vi "DevTests_Workbench.vi"() -> ()   [LabVIEW 2026]
uses:
  SDL3/Init/Init.lvlib
  SDL3/Video/Video.lvlib
  SDL3/Render/Render.lvlib
  SDL3/Pixels/PixelFormat--enum.ctl
  SDL3/Pixels/Pixels.lvlib
  SDL3/Render/TextureAccess-enum.ctl
  SDL3/Video/WindowFlags--ring.ctl
  SDL3/Init/InitFlags--ring.ctl
  SDL3/Timer/Timer.lvlib
  SDL3/Events/Events.lvlib
  SDL3/Video/WindowID--integer.ctl
  SDL3/Mouse/MouseID--integer.ctl
  SDL3/Mouse/Mouse.lvlib
  SDL3/Mouse/MouseButtonFlags--ring.ctl
  SDL3/Events/MouseMotionEventData--cluster.ctl
  SDL3/Rect/FPoint--cluster.ctl
  SDL3/Rect/Rect.lvlib
  SDL3/Video/GLAttr--enum.ctl
  SDL3/Rect/FRect--cluster.ctl
  SDL3/Blendmode/BlendMode--ring.ctl
  SDL3/Blendmode/Blendmode.lvlib
  SDL3/Keycode/Keycode--ring.ctl
  SDL3/Keycode/Keycode.lvlib
  SDL3/Video/DisplayID--integer.ctl
  SDL3/Video/DisplayMode--cluster.ctl
panel:
  out "Display Modes":T1[](array[typedef])
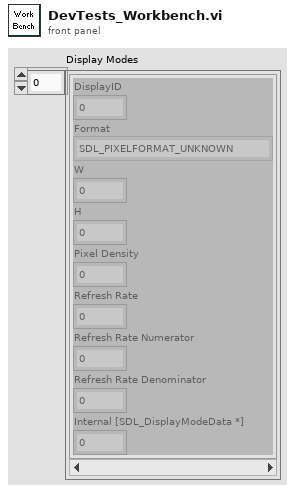
[diagram p1: front panel]
types:
  T1 = typedef "SDL3.lvlib/Video.lvlib/DisplayMode--cluster.ctl" = cluster{"DisplayID":T2, "Format":T3, "W":i32, "H":i32, "Pixel Density":sgl, "Refresh Rate":sgl, "Refresh Rate Numerator":i32, "Refresh Rate Denominator":i32, "Internal [SDL_DisplayModeData *]":i64}
  T2 = typedef "SDL3.lvlib/Video.lvlib/DisplayID--integer.ctl" = u32
  T3 = typedef "SDL3.lvlib/Pixels.lvlib/PixelFormat--enum.ctl" = enum32{"SDL_PIXELFORMAT_UNKNOWN", "SDL_PIXELFORMAT_INDEX1LSB", "SDL_PIXELFORMAT_INDEX1MSB", "SDL_PIXELFORMAT_INDEX2LSB", "SDL_PIXELFORMAT_INDEX2MSB", "SDL_PIXELFORMAT_INDEX4LSB", "SDL_PIXELFORMAT_INDEX4MSB", "SDL_PIXELFORMAT_INDEX8", "SDL_PIXELFORMAT_RGB332", "SDL_PIXELFORMAT_XRGB4444", "SDL_PIXELFORMAT_XBGR4444", "SDL_PIXELFORMAT_XRGB1555", "SDL_PIXELFORMAT_XBGR1555", "SDL_PIXELFORMAT_ARGB4444", "SDL_PIXELFORMAT_RGBA4444", "SDL_PIXELFORMAT_ABGR4444", "SDL_PIXELFORMAT_BGRA4444", "SDL_PIXELFORMAT_ARGB1555", "SDL_PIXELFORMAT_RGBA5551", "SDL_PIXELFORMAT_ABGR1555", "SDL_PIXELFORMAT_BGRA5551", "SDL_PIXELFORMAT_RGB565", "SDL_PIXELFORMAT_BGR565", "SDL_PIXELFORMAT_RGB24", "SDL_PIXELFORMAT_BGR24", "SDL_PIXELFORMAT_XRGB8888", "SDL_PIXELFORMAT_RGBX8888", "SDL_PIXELFORMAT_XBGR8888", "SDL_PIXELFORMAT_BGRX8888", "SDL_PIXELFORMAT_ARGB8888", "SDL_PIXELFORMAT_RGBA8888", "SDL_PIXELFORMAT_ABGR8888", "SDL_PIXELFORMAT_BGRA8888", "SDL_PIXELFORMAT_XRGB2101010", "SDL_PIXELFORMAT_XBGR2101010", "SDL_PIXELFORMAT_ARGB2101010", "SDL_PIXELFORMAT_ABGR2101010", "SDL_PIXELFORMAT_RGB48", "SDL_PIXELFORMAT_BGR48", "SDL_PIXELFORMAT_RGBA64", "SDL_PIXELFORMAT_ARGB64", "SDL_PIXELFORMAT_BGRA64", "SDL_PIXELFORMAT_ABGR64", "SDL_PIXELFORMAT_RGB48_FLOAT", "SDL_PIXELFORMAT_BGR48_FLOAT", "SDL_PIXELFORMAT_RGBA64_FLOAT", "SDL_PIXELFORMAT_ARGB64_FLOAT", "SDL_PIXELFORMAT_BGRA64_FLOAT", "SDL_PIXELFORMAT_ABGR64_FLOAT", "SDL_PIXELFORMAT_RGB96_FLOAT", "SDL_PIXELFORMAT_BGR96_FLOAT", "SDL_PIXELFORMAT_RGBA128_FLOAT", "SDL_PIXELFORMAT_ARGB128_FLOAT", "SDL_PIXELFORMAT_BGRA128_FLOAT", "SDL_PIXELFORMAT_ABGR128_FLOAT", "SDL_PIXELFORMAT_YV12", "SDL_PIXELFORMAT_IYUV", "SDL_PIXELFORMAT_YUY2", "SDL_PIXELFORMAT_UYVY", "SDL_PIXELFORMAT_YVYU", "SDL_PIXELFORMAT_NV12", "SDL_PIXELFORMAT_NV21", "SDL_PIXELFORMAT_P010", "SDL_PIXELFORMAT_EXTERNAL_OES"}
  T4 = typedef "SDL3.lvlib/Video.lvlib/WindowFlags--ring.ctl" = u64
  T5 = typedef "SDL3.lvlib/Blendmode.lvlib/BlendMode--ring.ctl" = u32
  T6 = typedef "SDL3.lvlib/Video.lvlib/GLAttr--enum.ctl" = enum32{"SDL_GL_RED_SIZE", "SDL_GL_GREEN_SIZE", "SDL_GL_BLUE_SIZE", "SDL_GL_ALPHA_SIZE", "SDL_GL_BUFFER_SIZE", "SDL_GL_DOUBLEBUFFER", "SDL_GL_DEPTH_SIZE", "SDL_GL_STENCIL_SIZE", "SDL_GL_ACCUM_RED_SIZE", "SDL_GL_ACCUM_GREEN_SIZE", "SDL_GL_ACCUM_BLUE_SIZE", "SDL_GL_ACCUM_ALPHA_SIZE", "SDL_GL_STEREO", "SDL_GL_MULTISAMPLEBUFFERS", "SDL_GL_MULTISAMPLESAMPLES", "SDL_GL_ACCELERATED_VISUAL", "SDL_GL_RETAINED_BACKING", "SDL_GL_CONTEXT_MAJOR_VERSION", "SDL_GL_CONTEXT_MINOR_VERSION", "SDL_GL_CONTEXT_FLAGS", "SDL_GL_CONTEXT_PROFILE_MASK", "SDL_GL_SHARE_WITH_CURRENT_CONTEXT", "SDL_GL_FRAMEBUFFER_SRGB_CAPABLE", "SDL_GL_CONTEXT_RELEASE_BEHAVIOR", "SDL_GL_CONTEXT_RESET_NOTIFICATION", "SDL_GL_CONTEXT_NO_ERROR", "SDL_GL_FLOATBUFFERS", "SDL_GL_EGL_PLATFORM"}
  T7 = enum32{"Invalid", "Standard", "Closed", "Hidden", "Minimized", "Maximized"}
  T8 = typedef "SDL3.lvlib/Events.lvlib/MouseMotionEventData--cluster.ctl" = cluster{"Timestamp":u64, "Window ID":T9, "Which":T10, "State":T11, "x":sgl, "y":sgl, "x Rel":sgl, "y Rel":sgl}
  T9 = typedef "SDL3.lvlib/Video.lvlib/WindowID--integer.ctl" = u32
  T10 = typedef "SDL3.lvlib/Mouse.lvlib/MouseID--integer.ctl" = u32
  T11 = typedef "SDL3.lvlib/Mouse.lvlib/MouseButtonFlags--ring.ctl" = u32
  T12 = typedef "SDL3.lvlib/Init.lvlib/InitFlags--ring.ctl" = u32
  T13 = typedef "SDL3.lvlib/Render.lvlib/TextureAccess-enum.ctl" = enum32{"SDL_TEXTUREACCESS_STATIC", "SDL_TEXTUREACCESS_STREAMING", "SDL_TEXTUREACCESS_TARGET"}
  T14 = typedef "SDL3.lvlib/Rect.lvlib/FPoint--cluster.ctl" = cluster{"x":sgl, "y":sgl}
  T15 = typedef "SDL3.lvlib/Rect.lvlib/FRect--cluster.ctl" = cluster{"x":sgl, "y":sgl, "w":sgl, "h":sgl}
  T16 = typedef "SDL3.lvlib/Events.lvlib/EventTypeData--enum.ctl" = enum16{"LV_NONE", "LV_UNSUPPORTED", "SDL_EVENT_QUIT", "SDL_EVENT_LOCALE_CHANGED", "SDL_EVENT_SYSTEM_THEME_CHANGED", "SDL_EVENT_DISPLAY_ORIENTATION", "SDL_EVENT_DISPLAY_ADDED", "SDL_EVENT_DISPLAY_REMOVED", "SDL_EVENT_DISPLAY_MOVED", "SDL_EVENT_DISPLAY_DESKTOP_MODE_CHANGED", "SDL_EVENT_DISPLAY_CURRENT_MODE_CHANGED", "SDL_EVENT_DISPLAY_CONTENT_SCALE_CHANGED", "SDL_EVENT_WINDOW_SHOWN", "SDL_EVENT_WINDOW_HIDDEN", "SDL_EVENT_WINDOW_EXPOSED", "SDL_EVENT_WINDOW_MOVED", "SDL_EVENT_WINDOW_RESIZED", "SDL_EVENT_WINDOW_PIXEL_SIZE_CHANGED", "SDL_EVENT_WINDOW_METAL_VIEW_RESIZED", "SDL_EVENT_WINDOW_MINIMIZED", "SDL_EVENT_WINDOW_MAXIMIZED", "SDL_EVENT_WINDOW_RESTORED", "SDL_EVENT_WINDOW_MOUSE_ENTER", "SDL_EVENT_WINDOW_MOUSE_LEAVE", "SDL_EVENT_WINDOW_FOCUS_GAINED", "SDL_EVENT_WINDOW_FOCUS_LOST", "SDL_EVENT_WINDOW_CLOSE_REQUESTED", "SDL_EVENT_WINDOW_HIT_TEST", "SDL_EVENT_WINDOW_ICCPROF_CHANGED", "SDL_EVENT_WINDOW_DISPLAY_CHANGED", "SDL_EVENT_WINDOW_DISPLAY_SCALE_CHANGED", "SDL_EVENT_WINDOW_SAFE_AREA_CHANGED", "SDL_EVENT_WINDOW_OCCLUDED", "SDL_EVENT_WINDOW_ENTER_FULLSCREEN", "SDL_EVENT_WINDOW_LEAVE_FULLSCREEN", "SDL_EVENT_WINDOW_DESTROYED", "SDL_EVENT_WINDOW_HDR_STATE_CHANGED", "SDL_EVENT_KEY_DOWN", "SDL_EVENT_KEY_UP", "SDL_EVENT_TEXT_EDITING", "SDL_EVENT_TEXT_INPUT", "SDL_EVENT_KEYMAP_CHANGED", "SDL_EVENT_KEYBOARD_ADDED", "SDL_EVENT_KEYBOARD_REMOVED", "SDL_EVENT_TEXT_EDITING_CANDIDATES", "SDL_EVENT_MOUSE_MOTION", "SDL_EVENT_MOUSE_BUTTON_DOWN", "SDL_EVENT_MOUSE_BUTTON_UP", "SDL_EVENT_MOUSE_WHEEL", "SDL_EVENT_MOUSE_ADDED", "SDL_EVENT_MOUSE_REMOVED", "SDL_EVENT_JOYSTICK_AXIS_MOTION", "SDL_EVENT_JOYSTICK_BALL_MOTION", "SDL_EVENT_JOYSTICK_HAT_MOTION", "SDL_EVENT_JOYSTICK_BUTTON_DOWN", "SDL_EVENT_JOYSTICK_BUTTON_UP", "SDL_EVENT_JOYSTICK_ADDED", "SDL_EVENT_JOYSTICK_REMOVED", "SDL_EVENT_JOYSTICK_BATTERY_UPDATED", "SDL_EVENT_JOYSTICK_UPDATE_COMPLETE", "SDL_EVENT_GAMEPAD_AXIS_MOTION", "SDL_EVENT_GAMEPAD_BUTTON_DOWN", "SDL_EVENT_GAMEPAD_BUTTON_UP", "SDL_EVENT_GAMEPAD_ADDED", "SDL_EVENT_GAMEPAD_REMOVED", "SDL_EVENT_GAMEPAD_REMAPPED", "SDL_EVENT_GAMEPAD_TOUCHPAD_DOWN", "SDL_EVENT_GAMEPAD_TOUCHPAD_MOTION", "SDL_EVENT_GAMEPAD_TOUCHPAD_UP", "SDL_EVENT_GAMEPAD_SENSOR_UPDATE", "SDL_EVENT_GAMEPAD_UPDATE_COMPLETE", "SDL_EVENT_GAMEPAD_STEAM_HANDLE_UPDATED", "SDL_EVENT_FINGER_DOWN", "SDL_EVENT_FINGER_UP", "SDL_EVENT_FINGER_MOTION", "SDL_EVENT_CLIPBOARD_UPDATE", "SDL_EVENT_DROP_FILE", "SDL_EVENT_DROP_TEXT", "SDL_EVENT_DROP_BEGIN", "SDL_EVENT_DROP_COMPLETE", "SDL_EVENT_DROP_POSITION", "SDL_EVENT_AUDIO_DEVICE_ADDED", "SDL_EVENT_AUDIO_DEVICE_REMOVED", "SDL_EVENT_AUDIO_DEVICE_FORMAT_CHANGED", "SDL_EVENT_SENSOR_UPDATE", "SDL_EVENT_PEN_PROXIMITY_IN", "SDL_EVENT_PEN_PROXIMITY_OUT", "SDL_EVENT_PEN_DOWN", "SDL_EVENT_PEN_UP", "SDL_EVENT_PEN_BUTTON_DOWN", "SDL_EVENT_PEN_BUTTON_UP", "SDL_EVENT_PEN_MOTION", "SDL_EVENT_PEN_AXIS", "SDL_EVENT_CAMERA_DEVICE_ADDED", "SDL_EVENT_CAMERA_DEVICE_REMOVED", "SDL_EVENT_CAMERA_DEVICE_APPROVED", "SDL_EVENT_CAMERA_DEVICE_DENIED", "SDL_EVENT_RENDER_TARGETS_RESET", "SDL_EVENT_RENDER_DEVICE_RESET", "SDL_EVENT_POLL_SENTINEL", "SDL_EVENT_USER"}
  T17 = typedef "SDL3.lvlib/Events.lvlib/MouseMotionEvent--cluster.ctl" = cluster{"Timestamp":u64, "Window ID":T9, "Which":T10, "State":T11, "x":sgl, "y":sgl, "x Rel":sgl, "y Rel":sgl}
  T18 = typedef "SDL3.lvlib/Keycode.lvlib/Keycode--ring.ctl" = u32
  T19 = typedef "SDL3.lvlib/Events.lvlib/KeyboardEventData--cluster.ctl" = cluster{"Timestamp":u64, "Window ID":T9, "Which":T20, "Scancode":T21, "Key":T18, "Mod":T22, "Raw":u16, "Down":bool, "Repeat":bool}
  T20 = typedef "SDL3.lvlib/Keyboard.lvlib/KeyboardID--integer.ctl" = u32
  T21 = typedef "SDL3.lvlib/Events.lvlib/Scancode--integer.ctl" = u32
  T22 = typedef "SDL3.lvlib/Keycode.lvlib/Keymod--ring.ctl" = u16
  T23 = typedef "SDL3.lvlib/Render.lvlib/Vertex--cluster.ctl" = cluster{"Position":T14, "Color":T24, "TexCoord":T14}
  T24 = typedef "SDL3.lvlib/Pixels.lvlib/FColor--cluster.ctl" = cluster{"r":sgl, "g":sgl, "b":sgl, "a":sgl}
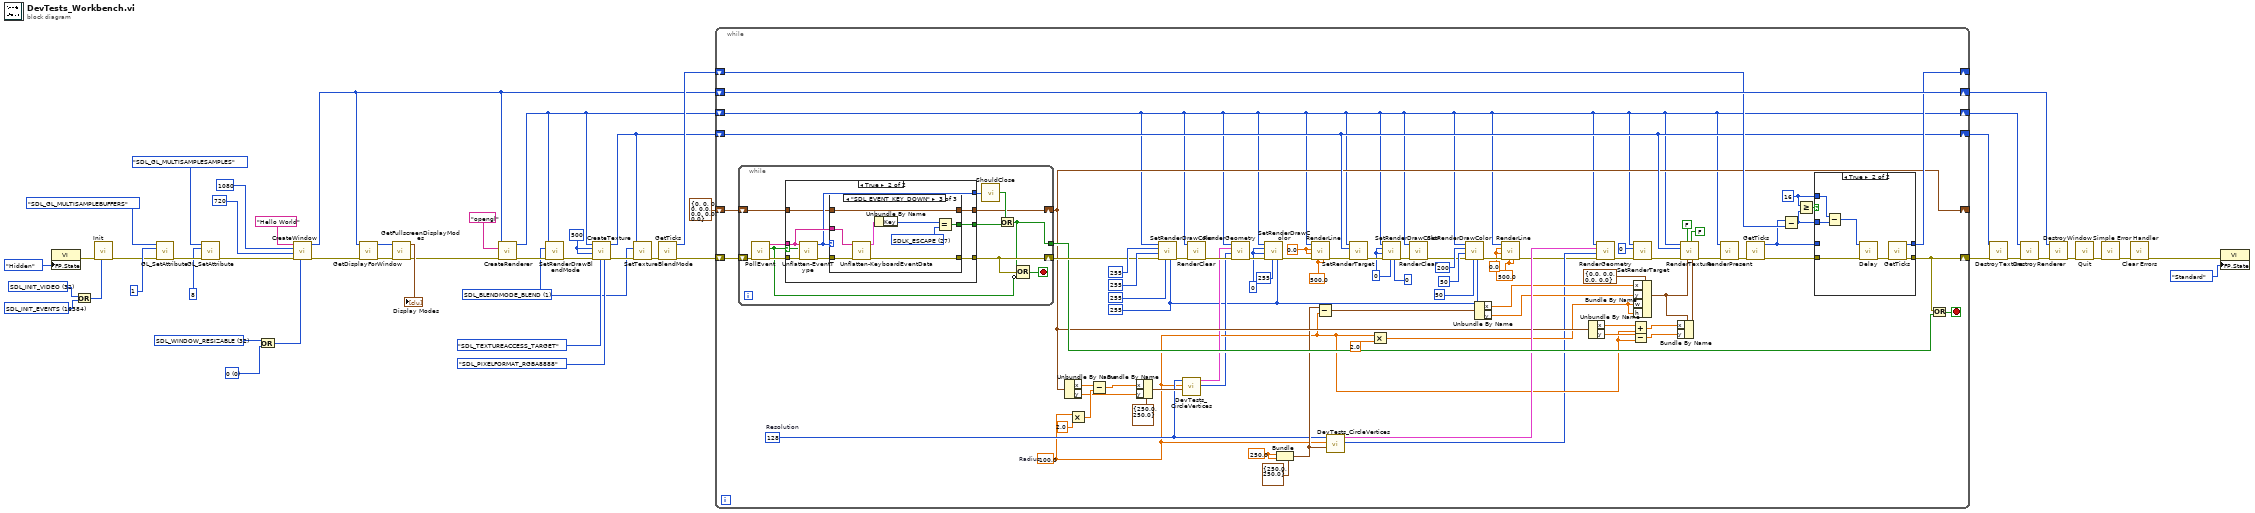
[diagram p0: block diagram]
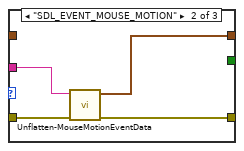
[diagram p4: hidden frame]
diagram:
  w10 = T4 0 items=["0"=0, "SDL_WINDOW_FULLSCREEN"=1, "SDL_WINDOW_OPENGL"=2, "SDL_WINDOW_OCCLUDED"=4, "SDL_WINDOW_HIDDEN"=8, "SDL_WINDOW_BORDERLESS"=16, "SDL_WINDOW_RESIZABLE"=32, "SDL_WINDOW_MINIMIZED"=64, "SDL_WINDOW_MAXIMIZED"=128, "SDL_WINDOW_MOUSE_GRABBED"=256, "SDL_WINDOW_INPUT_FOCUS"=512, "SDL_WINDOW_MOUSE_FOCUS"=1024, "SDL_WINDOW_EXTERNAL"=2048, "SDL_WINDOW_MODAL"=4096, "SDL_WINDOW_HIGH_PIXEL_DENSITY"=8192, "SDL_WINDOW_MOUSE_CAPTURE"=16384, "SDL_WINDOW_MOUSE_RELATIVE_MODE"=32768, "SDL_WINDOW_ALWAYS_ON_TOP"=65536, "SDL_WINDOW_UTILITY"=131072, "SDL_WINDOW_TOOLTIP"=262144, "SDL_WINDOW_POPUP_MENU"=524288, "SDL_WINDOW_KEYBOARD_GRABBED"=1048576, "SDL_WINDOW_VULKAN"=268435456, "SDL_WINDOW_METAL"=536870912, "SDL_WINDOW_TRANSPARENT"=1073741824, "SDL_WINDOW_NOT_FOCUSABLE"=2147483648] ("y")
  w7 = T5 1 items=["SDL_BLENDMODE_NONE"=0, "SDL_BLENDMODE_BLEND"=1, "SDL_BLENDMODE_BLEND_PREMULTIPLIED"=16, "SDL_BLENDMODE_ADD"=2, "SDL_BLENDMODE_ADD_PREMULTIPLIED"=32, "SDL_BLENDMODE_MOD"=4, "SDL_BLENDMODE_MUL"=8, "SDL_BLENDMODE_INVALID"=2147483647] ("Blend Mode")
  w25 = T12 16384 items=["NONE"=0, "SDL_INIT_AUDIO"=16, "SDL_INIT_VIDEO"=32, "SDL_INIT_JOYSTICK"=512, "SDL_INIT_HAPTIC"=4096, "SDL_INIT_GAMEPAD"=8192, "SDL_INIT_EVENTS"=16384, "SDL_INIT_SENSOR"=32768, "SDL_INIT_CAMER"=65536] ("y")
  w29 = T12 32 items=["NONE"=0, "SDL_INIT_AUDIO"=16, "SDL_INIT_VIDEO"=32, "SDL_INIT_JOYSTICK"=512, "SDL_INIT_HAPTIC"=4096, "SDL_INIT_GAMEPAD"=8192, "SDL_INIT_EVENTS"=16384, "SDL_INIT_SENSOR"=32768, "SDL_INIT_CAMER"=65536] ("InitFlags")
  w43 = 500 ("w")
  w47 = T4 32 items=["0"=0, "SDL_WINDOW_FULLSCREEN"=1, "SDL_WINDOW_OPENGL"=2, "SDL_WINDOW_OCCLUDED"=4, "SDL_WINDOW_HIDDEN"=8, "SDL_WINDOW_BORDERLESS"=16, "SDL_WINDOW_RESIZABLE"=32, "SDL_WINDOW_MINIMIZED"=64, "SDL_WINDOW_MAXIMIZED"=128, "SDL_WINDOW_MOUSE_GRABBED"=256, "SDL_WINDOW_INPUT_FOCUS"=512, "SDL_WINDOW_MOUSE_FOCUS"=1024, "SDL_WINDOW_EXTERNAL"=2048, "SDL_WINDOW_MODAL"=4096, "SDL_WINDOW_HIGH_PIXEL_DENSITY"=8192, "SDL_WINDOW_MOUSE_CAPTURE"=16384, "SDL_WINDOW_MOUSE_RELATIVE_MODE"=32768, "SDL_WINDOW_ALWAYS_ON_TOP"=65536, "SDL_WINDOW_UTILITY"=131072, "SDL_WINDOW_TOOLTIP"=262144, "SDL_WINDOW_POPUP_MENU"=524288, "SDL_WINDOW_KEYBOARD_GRABBED"=1048576, "SDL_WINDOW_VULKAN"=268435456, "SDL_WINDOW_METAL"=536870912, "SDL_WINDOW_TRANSPARENT"=1073741824, "SDL_WINDOW_NOT_FOCUSABLE"=2147483648] ("flags (0)")
  n1 = property class="VI"("FP.State"=T7."Hidden" ("Front Panel Window:State")) -> (error out=w34:errorcluster)  [unwired: 2 in, 1 out]
  n2 = Or(x=w29, y=w25) -> (x .or. y?=w26:T12)
  n3 = call "Init.vi"("InitFlags"=w26, "No Error"=w34) -> ("error out"=w13:errorcluster)  [unwired: 9 in]
  n4 = call "GL_SetAttribute.vi"("No Error"=w13, "Value"=1, "GL Attribute"=GLAttr--enum."SDL_GL_MULTISAMPLEBUFFERS") -> ("Error Out"=w21:errorcluster)  [unwired: 8 in]
  n5 = call "GL_SetAttribute.vi"("No Error"=w21, "Value"=8, "GL Attribute"=GLAttr--enum."SDL_GL_MULTISAMPLESAMPLES") -> ("Error Out"=w22:errorcluster)  [unwired: 8 in]
  n6 = Compound Arithmetic op=OR(w47, w10) -> (w11:T4)
  n7 = call "CreateWindow.vi"("Flags (0)"=w11, "No Error"=w22, "h"=720, "w"=1080, "Title"="Hello World" ("title")) -> ("Error Out"=w6:errorcluster, "Window [SDL_Window *]"=w5:i64)  [unwired: 5 in]
  n8 = call "GetDisplayForWindow.vi"("No Error"=w6, "Window [SDL_Window *]"=w5) -> ("Error Out"=w4:errorcluster, "DisplayID"=w3:T2)  [unwired: 8 in]
  n9 = call "GetFullscreenDisplayModes.vi"("No Error"=w4, "DisplayID"=w3) -> ("Error Out"=w1:errorcluster, "Display Modes"=→"Display Modes":T1[])  [unwired: 8 in]
  n10 = call "CreateRenderer.vi"("No Error"=w1, "Name (\"\": NULL)"="opengl" ("Name (\"\": NULL)"), "Window [SDL_Window *]"=w5) -> ("Error Out"=w44:errorcluster, "Renderer [SDL_Renderer *]"=w8:i64)  [unwired: 7 in]
  n11 = call "SetRenderDrawBlendMode.vi"("No Error"=w44, "Blend Mode"=w7, "Renderer [SDL_Renderer *]"=w8) -> ("error out"=w9:errorcluster)  [unwired: 8 in]
  n12 = call "CreateTexture.vi"("Pixel Format"=PixelFormat--enum."SDL_PIXELFORMAT_RGBA8888" ("pixel_format"), "Texture Access"=TextureAccess-enum."SDL_TEXTUREACCESS_TARGET" ("texture_access"), "No Error"=w9, "h"=w43, "w"=w43, "Renderer [SDL_Renderer *]"=w8) -> ("error out"=w16:errorcluster, "Texture [SDL_Texture *]"=w14:i64)  [unwired: 4 in]
  n13 = call "SetTextureBlendMode.vi"("No Error"=w16, "Blend Mode"=w7, "Texture [SDL_Texture *]"=w14) -> ("error out"=w15:errorcluster)  [unwired: 8 in]
  n14 = call "GetTicks.vi"("No Error"=w15) -> ("error out"=w28:errorcluster, "Ticks [ms]"=w27:u64)  [unwired: 9 in]
  n15 = while {
    shift-right: [w98] -> w37
    shift-left: w14 -> [w98]
    shift-right: [w53] -> w38
    shift-left: w8 -> [w53]
    shift-right: [w126] -> w39
    shift-left: w5 -> [w126]
    shift-right: [w100] -> w46
    shift-left: w28 -> [w106]
    shift-right: [w114] -> _
    shift-left: w27 -> [w111]
    shift-right: [w97] -> _
    shift-left: T8 {"Timestamp"=0, "Window ID"=0, "Which"=0, "State"=0, "x"=0.0, "y"=0.0, "x Rel"=0.0, "y Rel"=0.0} ("MouseMotionEvent") -> [w105]
    stop <- w101 stop-if-true
    w51 = sgl 500.0 ("X2")
    w52 = sgl 0.0 ("X1")
    w57 = u8 0 ("R")
    w61 = sgl 0.0 ("X1")
    w62 = sgl 500.0 ("X2")
    w66 = u8 0 ("r")
    w84 = sgl 250.0 ("x")
    w71 = sgl 100.0  # Radius
    w77 = 128  # Resolution
    w110 = u64 16
    w58 = u8 255 ("a")
    n16 = while {
      shift-right: [w129] -> w104
      shift-left: w106 -> [w138]
      tunnel: [w128] -> w102
      shift-right: [w131] -> w97
      shift-left: w105 -> [w130]
      stop <- w137 stop-if-true
      n17 = call "PollEvent.vi"("No Error"=w138) -> ("error out"=w136:errorcluster, "Event Occured?"=w134:bool, "Event Binary Data"=w135:string)  [unwired: 8 in]
      n18 = case shown="True" w134 {
        tunnel: w136 -> [w140 w148]
        tunnel: w135 -> [_ w147]
        tunnel: [w140 w144] -> w129
        tunnel: [_ w146] -> w133
        tunnel: [w139 w143] -> w131
        tunnel: w130 -> [w139 w142]
        tunnel: [_ w141] -> w127
        frame False {
        }
        frame True {
          n19 = call "Unflatten-EventType.vi"("error in (no error)"=w148, "Event Binary Data In"=w147) -> ("error out"=w145:errorcluster, "EventType"=w146:T16)  [unwired: 8 in]
          n20 = case shown="\"SDL_EVENT_KEY_DOWN\"" w146 {
            tunnel: w147 -> [_ w153 w160]
            tunnel: w145 -> [w150 w154 w161]
            tunnel: [w150 w152 w159] -> w144
            tunnel: [w149 w151 w162] -> w143
            tunnel: w142 -> [w149 _ w162]
            tunnel: [_ _ w155] -> w141
            frame Default {
            }
            frame "SDL_EVENT_MOUSE_MOTION" {
              n21 = call "Unflatten-MouseMotionEventData.vi"("error in (no error)"=w154, "Event Binary Data"=w153) -> ("error out"=w152:errorcluster, "Event Data"=w151:T17)  [unwired: 8 in]
            }
            frame "SDL_EVENT_KEY_DOWN" {
              w156 = T18 27 items=["SDLK_SCANCODE_MASK"=1073741824, "SDLK_UNKNOWN"=0, "SDLK_RETURN"=13, "SDLK_ESCAPE"=27, "SDLK_BACKSPACE"=8, "SDLK_TAB"=9, "SDLK_SPACE"=32, "SDLK_EXCLAIM"=33, "SDLK_DBLAPOSTROPHE"=34, "SDLK_HASH"=35, "SDLK_DOLLAR"=36, "SDLK_PERCENT"=37, "SDLK_AMPERSAND"=38, "SDLK_APOSTROPHE"=39, "SDLK_LEFTPAREN"=40, "SDLK_RIGHTPAREN"=41, "SDLK_ASTERISK"=42, "SDLK_PLUS"=43, "SDLK_COMMA"=44, "SDLK_MINUS"=45, "SDLK_PERIOD"=46, "SDLK_SLASH"=47, "SDLK_0"=48, "SDLK_1"=49, "SDLK_2"=50, "SDLK_3"=51, "SDLK_4"=52, "SDLK_5"=53, "SDLK_6"=54, "SDLK_7"=55, "SDLK_8"=56, "SDLK_9"=57, "SDLK_COLON"=58, "SDLK_SEMICOLON"=59, "SDLK_LESS"=60, "SDLK_EQUALS"=61, "SDLK_GREATER"=62, "SDLK_QUESTION"=63, "SDLK_AT"=64, "SDLK_LEFTBRACKET"=91, "SDLK_BACKSLASH"=92, "SDLK_RIGHTBRACKET"=93, "SDLK_CARET"=94, "SDLK_UNDERSCORE"=95, "SDLK_GRAVE"=96, "SDLK_A"=97, "SDLK_B"=98, "SDLK_C"=99, "SDLK_D"=100, "SDLK_E"=101, "SDLK_F"=102, "SDLK_G"=103, "SDLK_H"=104, "SDLK_I"=105, "SDLK_J"=106, "SDLK_K"=107, "SDLK_L"=108, "SDLK_M"=109, "SDLK_N"=110, "SDLK_O"=111, "SDLK_P"=112, "SDLK_Q"=113, "SDLK_R"=114, "SDLK_S"=115, "SDLK_T"=116, "SDLK_U"=117, "SDLK_V"=118, "SDLK_W"=119, "SDLK_X"=120, "SDLK_Y"=121, "SDLK_Z"=122, "SDLK_LEFTBRACE"=123, "SDLK_PIPE"=124, "SDLK_RIGHTBRACE"=125, "SDLK_TILDE"=126, "SDLK_DELETE"=127, "SDLK_PLUSMINUS"=177, "SDLK_CAPSLOCK"=1073741881, "SDLK_F1"=1073741882, "SDLK_F2"=1073741883, "SDLK_F3"=1073741884, "SDLK_F4"=1073741885, "SDLK_F5"=1073741886, "SDLK_F6"=1073741887, "SDLK_F7"=1073741888, "SDLK_F8"=1073741889, "SDLK_F9"=1073741890, "SDLK_F10"=1073741891, "SDLK_F11"=1073741892, "SDLK_F12"=1073741893, "SDLK_PRINTSCREEN"=1073741894, "SDLK_SCROLLLOCK"=1073741895, "SDLK_PAUSE"=1073741896, "SDLK_INSERT"=1073741897, "SDLK_HOME"=1073741898, "SDLK_PAGEUP"=1073741899, "SDLK_END"=1073741901, "SDLK_PAGEDOWN"=1073741902, "SDLK_RIGHT"=1073741903, "SDLK_LEFT"=1073741904, "SDLK_DOWN"=1073741905, "SDLK_UP"=1073741906, "SDLK_NUMLOCKCLEAR"=1073741907, "SDLK_KP_DIVIDE"=1073741908, "SDLK_KP_MULTIPLY"=1073741909, "SDLK_KP_MINUS"=1073741910, "SDLK_KP_PLUS"=1073741911, "SDLK_KP_ENTER"=1073741912, "SDLK_KP_1"=1073741913, "SDLK_KP_2"=1073741914, "SDLK_KP_3"=1073741915, "SDLK_KP_4"=1073741916, "SDLK_KP_5"=1073741917, "SDLK_KP_6"=1073741918, "SDLK_KP_7"=1073741919, "SDLK_KP_8"=1073741920, "SDLK_KP_9"=1073741921, "SDLK_KP_0"=1073741922, "SDLK_KP_PERIOD"=1073741923, "SDLK_APPLICATION"=1073741925, "SDLK_POWER"=1073741926, "SDLK_KP_EQUALS"=1073741927, "SDLK_F13"=1073741928, "SDLK_F14"=1073741929, "SDLK_F15"=1073741930, "SDLK_F16"=1073741931, "SDLK_F17"=1073741932, "SDLK_F18"=1073741933, "SDLK_F19"=1073741934, "SDLK_F20"=1073741935, "SDLK_F21"=1073741936, "SDLK_F22"=1073741937, "SDLK_F23"=1073741938, "SDLK_F24"=1073741939, "SDLK_EXECUTE"=1073741940, "SDLK_HELP"=1073741941, "SDLK_MENU"=1073741942, "SDLK_SELECT"=1073741943, "SDLK_STOP"=1073741944, "SDLK_AGAIN"=1073741945, "SDLK_UNDO"=1073741946, "SDLK_CUT"=1073741947, "SDLK_COPY"=1073741948, "SDLK_PASTE"=1073741949, "SDLK_FIND"=1073741950, "SDLK_MUTE"=1073741951, "SDLK_VOLUMEUP"=1073741952, "SDLK_VOLUMEDOWN"=1073741953, "SDLK_KP_COMMA"=1073741957, "SDLK_KP_EQUALSAS400"=1073741958, "SDLK_ALTERASE"=1073741977, "SDLK_SYSREQ"=1073741978, "SDLK_CANCEL"=1073741979, "SDLK_CLEAR"=1073741980, "SDLK_PRIOR"=1073741981, "SDLK_RETURN2"=1073741982, "SDLK_SEPARATOR"=1073741983, "SDLK_OUT"=1073741984, "SDLK_OPER"=1073741985, "SDLK_CLEARAGAIN"=1073741986, "SDLK_CRSEL"=1073741987, "SDLK_EXSEL"=1073741988, "SDLK_KP_00"=1073742000, "SDLK_KP_000"=1073742001, "SDLK_THOUSANDSSEPARATOR"=1073742002, "SDLK_DECIMALSEPARATOR"=1073742003, "SDLK_CURRENCYUNIT"=1073742004, "SDLK_CURRENCYSUBUNIT"=1073742005, "SDLK_KP_LEFTPAREN"=1073742006, "SDLK_KP_RIGHTPAREN"=1073742007, "SDLK_KP_LEFTBRACE"=1073742008, "SDLK_KP_RIGHTBRACE"=1073742009, "SDLK_KP_TAB"=1073742010, "SDLK_KP_BACKSPACE"=1073742011, "SDLK_KP_A"=1073742012, "SDLK_KP_B"=1073742013, "SDLK_KP_C"=1073742014, "SDLK_KP_D"=1073742015, "SDLK_KP_E"=1073742016, "SDLK_KP_F"=1073742017, "SDLK_KP_XOR"=1073742018, "SDLK_KP_POWER"=1073742019, "SDLK_KP_PERCENT"=1073742020, "SDLK_KP_LESS"=1073742021, "SDLK_KP_GREATER"=1073742022, "SDLK_KP_AMPERSAND"=1073742023, "SDLK_KP_DBLAMPERSAND"=1073742024, "SDLK_KP_VERTICALBAR"=1073742025, "SDLK_KP_DBLVERTICALBAR"=1073742026, "SDLK_KP_COLON"=1073742027, "SDLK_KP_HASH"=1073742028, "SDLK_KP_SPACE"=1073742029, "SDLK_KP_AT"=1073742030, "SDLK_KP_EXCLAM"=1073742031, "SDLK_KP_MEMSTORE"=1073742032, "SDLK_KP_MEMRECALL"=1073742033, "SDLK_KP_MEMCLEAR"=1073742034, "SDLK_KP_MEMADD"=1073742035, "SDLK_KP_MEMSUBTRACT"=1073742036, "SDLK_KP_MEMMULTIPLY"=1073742037, "SDLK_KP_MEMDIVIDE"=1073742038, "SDLK_KP_PLUSMINUS"=1073742039, "SDLK_KP_CLEAR"=1073742040, "SDLK_KP_CLEARENTRY"=1073742041, "SDLK_KP_BINARY"=1073742042, "SDLK_KP_OCTAL"=1073742043, "SDLK_KP_DECIMAL"=1073742044, "SDLK_KP_HEXADECIMAL"=1073742045, "SDLK_LCTRL"=1073742048, "SDLK_LSHIFT"=1073742049, "SDLK_LALT"=1073742050, "SDLK_LGUI"=1073742051, "SDLK_RCTRL"=1073742052, "SDLK_RSHIFT"=1073742053, "SDLK_RALT"=1073742054, "SDLK_RGUI"=1073742055, "SDLK_MODE"=1073742081, "SDLK_SLEEP"=1073742082, "SDLK_WAKE"=1073742083, "SDLK_CHANNEL_INCREMENT"=1073742084, "SDLK_CHANNEL_DECREMENT"=1073742085, "SDLK_MEDIA_PLAY"=1073742086, "SDLK_MEDIA_PAUSE"=1073742087, "SDLK_MEDIA_RECORD"=1073742088, "SDLK_MEDIA_FAST_FORWARD"=1073742089, "SDLK_MEDIA_REWIND"=1073742090, "SDLK_MEDIA_NEXT_TRACK"=1073742091, "SDLK_MEDIA_PREVIOUS_TRACK"=1073742092, "SDLK_MEDIA_STOP"=1073742093, "SDLK_MEDIA_EJECT"=1073742094, "SDLK_MEDIA_PLAY_PAUSE"=1073742095, "SDLK_MEDIA_SELECT"=1073742096, "SDLK_AC_NEW"=1073742097, "SDLK_AC_OPEN"=1073742098, "SDLK_AC_CLOSE"=1073742099, "SDLK_AC_EXIT"=1073742100, "SDLK_AC_SAVE"=1073742101, "SDLK_AC_PRINT"=1073742102, "SDLK_AC_PROPERTIES"=1073742103, "SDLK_AC_SEARCH"=1073742104, "SDLK_AC_HOME"=1073742105, "SDLK_AC_BACK"=1073742106, "SDLK_AC_FORWARD"=1073742107, "SDLK_AC_STOP"=1073742108, "SDLK_AC_REFRESH"=1073742109, "SDLK_AC_BOOKMARKS"=1073742110, "SDLK_SOFTLEFT"=1073742111, "SDLK_SOFTRIGHT"=1073742112, "SDLK_CALL"=1073742113, "SDLK_ENDCALL"=1073742114] ("y")
              n22 = call "Unflatten-KeyboardEventData.vi"("error in (no error)"=w161, "Event Binary Data"=w160) -> ("error out"=w159:errorcluster, "Event Data"=w158:T19)  [unwired: 8 in]
              n23 = Unbundle By Name(w158) -> ("Key"=w157:T18)
              n24 = Equal?(x=w157, y=w156) -> (x = y?=w155:bool)
            }
          }
        }
      }
      n25 = call "ShouldClose.vi"("EventType"=w133) -> ("Close?"=w132:bool)
      n26 = Or(x=w132, y=w127) -> (x .or. y?=w128:bool)
      n27 = Compound Arithmetic op=OR(w128, w129, invert w134) -> (w137:bool)
    }
    n28 = Unbundle By Name(w97) -> ("x"=w79:sgl, "y"=w72:sgl)
    n29 = Multiply(x=w71, y=sgl 2.0) -> (x*y=w74:sgl)
    n30 = Subtract(x=w79, y=w74) -> (x-y=w75:sgl)
    n31 = Bundle By Name(cluster=T14 {"x"=250.0, "y"=250.0} ("Center"), "x"=w75, "y"=w72) -> (w78:T14)
    n32 = call "SetRenderDrawColor.vi"("a"=w58, "b"=u8 255, "No Error"=w104, "g"=u8 255, "r"=u8 255, "Renderer [SDL_Renderer *]"=w53) -> ("error out"=w123:errorcluster)  [unwired: 5 in]
    n33 = call "DevTests_CircleVertices.vi"("Center"=w78, "Radius"=w71, "Quality"=w77) -> ("Draw Order"=w70:i32[], "Vertices"=w76:T23[])  [unwired: 7 in]
    n34 = call "RenderClear.vi"("No Error"=w123, "Renderer [SDL_Renderer *]"=w53) -> ("error out"=w81:errorcluster)  [unwired: 9 in]
    n35 = call "RenderGeometry.vi"("No Error"=w81, "Indices (Empty)"=w70, "Vertices"=w76, "Renderer [SDL_Renderer *]"=w53) -> ("error out"=w59:errorcluster)  [unwired: 7 in]
    n36 = call "SetRenderDrawColor.vi"("a"=w58, "b"=u8 255 ("B"), "No Error"=w59, "g"=w57, "r"=w57, "Renderer [SDL_Renderer *]"=w53) -> ("error out"=w55:errorcluster)  [unwired: 5 in]
    n37 = Bundle(cluster=T14 {"x"=250.0, "y"=250.0} ("Center"), "x"=w84, "y"=w84) -> (w83:T14)
    n38 = call "RenderLine.vi"("y2"=w62, "x2"=w62, "No Error"=w55, "y1"=w61, "x1"=w61, "Renderer [SDL_Renderer *]"=w53) -> ("error out"=w60:errorcluster)  [unwired: 5 in]
    n39 = Subtract(x=w83, y=w71) -> (x-y=w90:T14)
    n40 = call "DevTests_CircleVertices.vi"("Center"=w83, "Radius"=w71, "Quality"=w77) -> ("Draw Order"=w69:i32[], "Vertices"=w99:T23[])  [unwired: 7 in]
    n41 = call "SetRenderTarget.vi"("No Error"=w60, "Texture [SDL_Texture *]"=w98, "Renderer [SDL_Renderer *]"=w53) -> ("error out"=w68:errorcluster)  [unwired: 8 in]
    n42 = Multiply(x=w71, y=sgl 2.0) -> (x*y=w85:sgl)
    n43 = call "SetRenderDrawColor.vi"("a"=u8 0 ("A"), "b"=w66, "No Error"=w68, "g"=w66, "r"=w66, "Renderer [SDL_Renderer *]"=w53) -> ("error out"=w67:errorcluster)  [unwired: 5 in]
    n44 = call "RenderClear.vi"("No Error"=w67, "Renderer [SDL_Renderer *]"=w53) -> ("error out"=w103:errorcluster)  [unwired: 9 in]
    n45 = call "SetRenderDrawColor.vi"("a"=w58, "b"=u8 50, "No Error"=w103, "g"=u8 50, "r"=u8 200, "Renderer [SDL_Renderer *]"=w53) -> ("error out"=w54:errorcluster)  [unwired: 5 in]
    n46 = Unbundle By Name(w90) -> ("x"=w89:sgl, "y"=w88:sgl)
    n47 = call "RenderLine.vi"("y2"=w51, "x2"=w51, "No Error"=w54, "y1"=w52, "x1"=w52, "Renderer [SDL_Renderer *]"=w53) -> ("error out"=w50:errorcluster)  [unwired: 5 in]
    n48 = Unbundle By Name(w97) -> ("x"=w95:sgl, "y"=w94:sgl)
    n49 = call "RenderGeometry.vi"("No Error"=w50, "Indices (Empty)"=w69, "Vertices"=w99, "Renderer [SDL_Renderer *]"=w53) -> ("error out"=w115:errorcluster)  [unwired: 7 in]
    n50 = Add(x=w95, y=w71) -> (x+y=w93:sgl)
    n51 = Subtract(x=w94, y=w71) -> (x-y=w92:sgl)
    n52 = Bundle By Name(cluster=T15 {"x"=0.0, "y"=0.0, "w"=0.0, "h"=0.0} ("Srcrect"), "x"=w89, "y"=w88, "w"=w85, "h"=w85) -> (w87:T15)
    n53 = call "SetRenderTarget.vi"("No Error"=w115, "Texture [SDL_Texture *]"=i64 0 ("texture [SDL_Texture *]"), "Renderer [SDL_Renderer *]"=w53) -> ("error out"=w124:errorcluster)  [unwired: 8 in]
    n54 = Bundle By Name(cluster=w87, "x"=w93, "y"=w92) -> (w96:T15)
    n55 = call "RenderTexture.vi"("Dstrect"=w96, "Entire Rendering Target (F)"=FALSE, "Srcrect"=w87, "Entire Texture (F)"=FALSE, "No Error"=w124, "Texture [SDL_Texture *]"=w98, "Renderer [SDL_Renderer *]"=w53) -> ("error out"=w125:errorcluster)  [unwired: 4 in]
    n56 = call "RenderPresent.vi"("No Error"=w125, "Renderer [SDL_Renderer *]"=w53) -> ("error out"=w113:errorcluster)  [unwired: 9 in]
    n57 = call "GetTicks.vi"("No Error"=w113) -> ("error out"=w112:errorcluster, "Ticks [ms]"=w107:u64)  [unwired: 9 in]
    n58 = Subtract(x=w107, y=w111) -> (x-y=w109:u64)
    n59 = Greater Or Equal?(x=w110, y=w109) -> (x >= y?=w108:bool)
    n60 = case shown="True" w108 {
      tunnel: [w163 w171] -> w100
      tunnel: [w164 w170] -> w114
      tunnel: w112 -> [w163 w169]
      tunnel: w110 -> [_ w168]
      tunnel: w109 -> [_ w167]
      tunnel: w107 -> [w164 _]
      frame False {
      }
      frame True {
        n61 = Subtract(x=w168, y=w167) -> (x-y=w165:u64)
        n62 = call "Delay.vi"("No Error"=w169, "ms"=w165) -> ("error out"=w166:errorcluster)  [unwired: 9 in]
        n63 = call "GetTicks.vi"("No Error"=w166) -> ("error out"=w171:errorcluster, "Ticks [ms]"=w170:u64)  [unwired: 9 in]
      }
    }
    n64 = Or(x=w100, y=w102) -> (x .or. y?=w101:bool)
  }
  n65 = call "DestroyTexture.vi"("No Error"=w46, "Texture [SDL_Texture *]"=w37) -> ("error out"=w40:errorcluster)  [unwired: 9 in]
  n66 = call "DestroyRenderer.vi"("No Error"=w40, "Rrenderer [SDL_Renderer *]"=w38) -> ("error out"=w45:errorcluster)  [unwired: 9 in]
  n67 = call "DestroyWindow.vi"("No Error"=w45, "Window [SDL_Window*]"=w39) -> ("Error Out"=w49:errorcluster)  [unwired: 9 in]
  n68 = call "Quit.vi"("No Error"=w49) -> ("error out"=w32:errorcluster)  [unwired: 10 in]
  n69 = call <vilib>:"Simple Error Handler.vi"("error in (no error)"=w32) -> ("error out"=w31:errorcluster)  [unwired: 4 in, 4 out]
  n70 = call <vilib>:"Clear Errors.vi"("error in (no error)"=w31) -> ("error out"=w30:errorcluster)  [unwired: 5 in, 1 out]
  n71 = property class="VI"(error in=w30, "FP.State"=T7."Standard" ("Front Panel Window:State")) -> ()  [unwired: 1 in, 2 out]
